vi "Cycle_Diag_Table_Read_TL24.vi"(7 "ERD Data In":T3[](array[typedef]) {"ERD Number" format="%.0x"}, 11 "error in (no error)":errorcluster) -> (2 "Cycle Buffer Status":T2, 3 "Diag Cycle String Out":string[][](array[string]), 8 "Cycle  Diag Array Out":T1[](array[typedef]), 15 "error out":errorcluster)   [LabVIEW 2016]
uses:
  Common/LabVIEW GEA2 Toolkit/LabVIEW_GEA2_Toolkit.lvlibp/type defs/ERD Read Data Out.ctl
  type defs/Cycle_Diag_Buffer_Status.ctl
  type defs/Cycle_Diag.ctl
  Common/LabVIEW GEA2 Toolkit/LabVIEW_GEA2_Toolkit.lvlibp
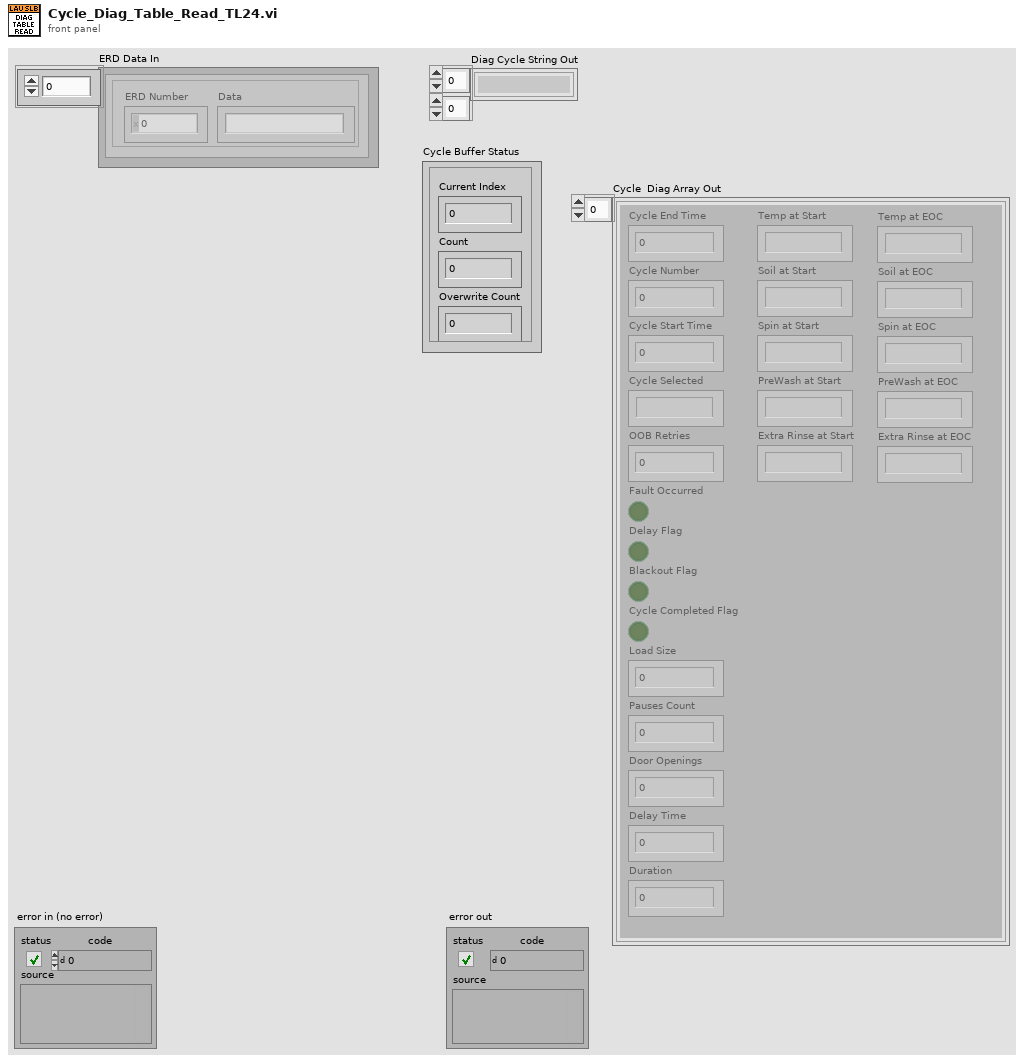
[diagram p1: front panel]
types:
  T1 = typedef "Cycle_Diag.ctl" = cluster{"Cycle End Time":u32, "Cycle Number":u32, "Cycle Start Time":u32, "OOB Retries":u8, "Temp at Start":string, "Soil at Start":string, "PreWash at Start":string, "Extra Rinse at Start":string, "Pauses Count":u8, "Fault Occurred":bool, "Delay Flag":bool, "Blackout Flag":bool, "Cycle Completed Flag":bool, "Temp at EOC":string, "Soil at EOC":string, "PreWash at EOC":string, "Extra Rinse at EOC":string, "Load Size":u8, "Door Openings":u8, "Cycle Selected":string, "Spin at Start":string, "Spin at EOC":string, "Delay Time":u16, "Duration":dbl}
  T2 = typedef "Cycle_Diag_Buffer_Status.ctl" = cluster{"Current Index":u16, "Count":u16, "Overwrite Count":u16}
  T3 = typedef "LabVIEW_GEA2_Toolkit.lvlibp/ERD Read Data Out.ctl" = cluster{"ERD Number":u16, "Data":string}
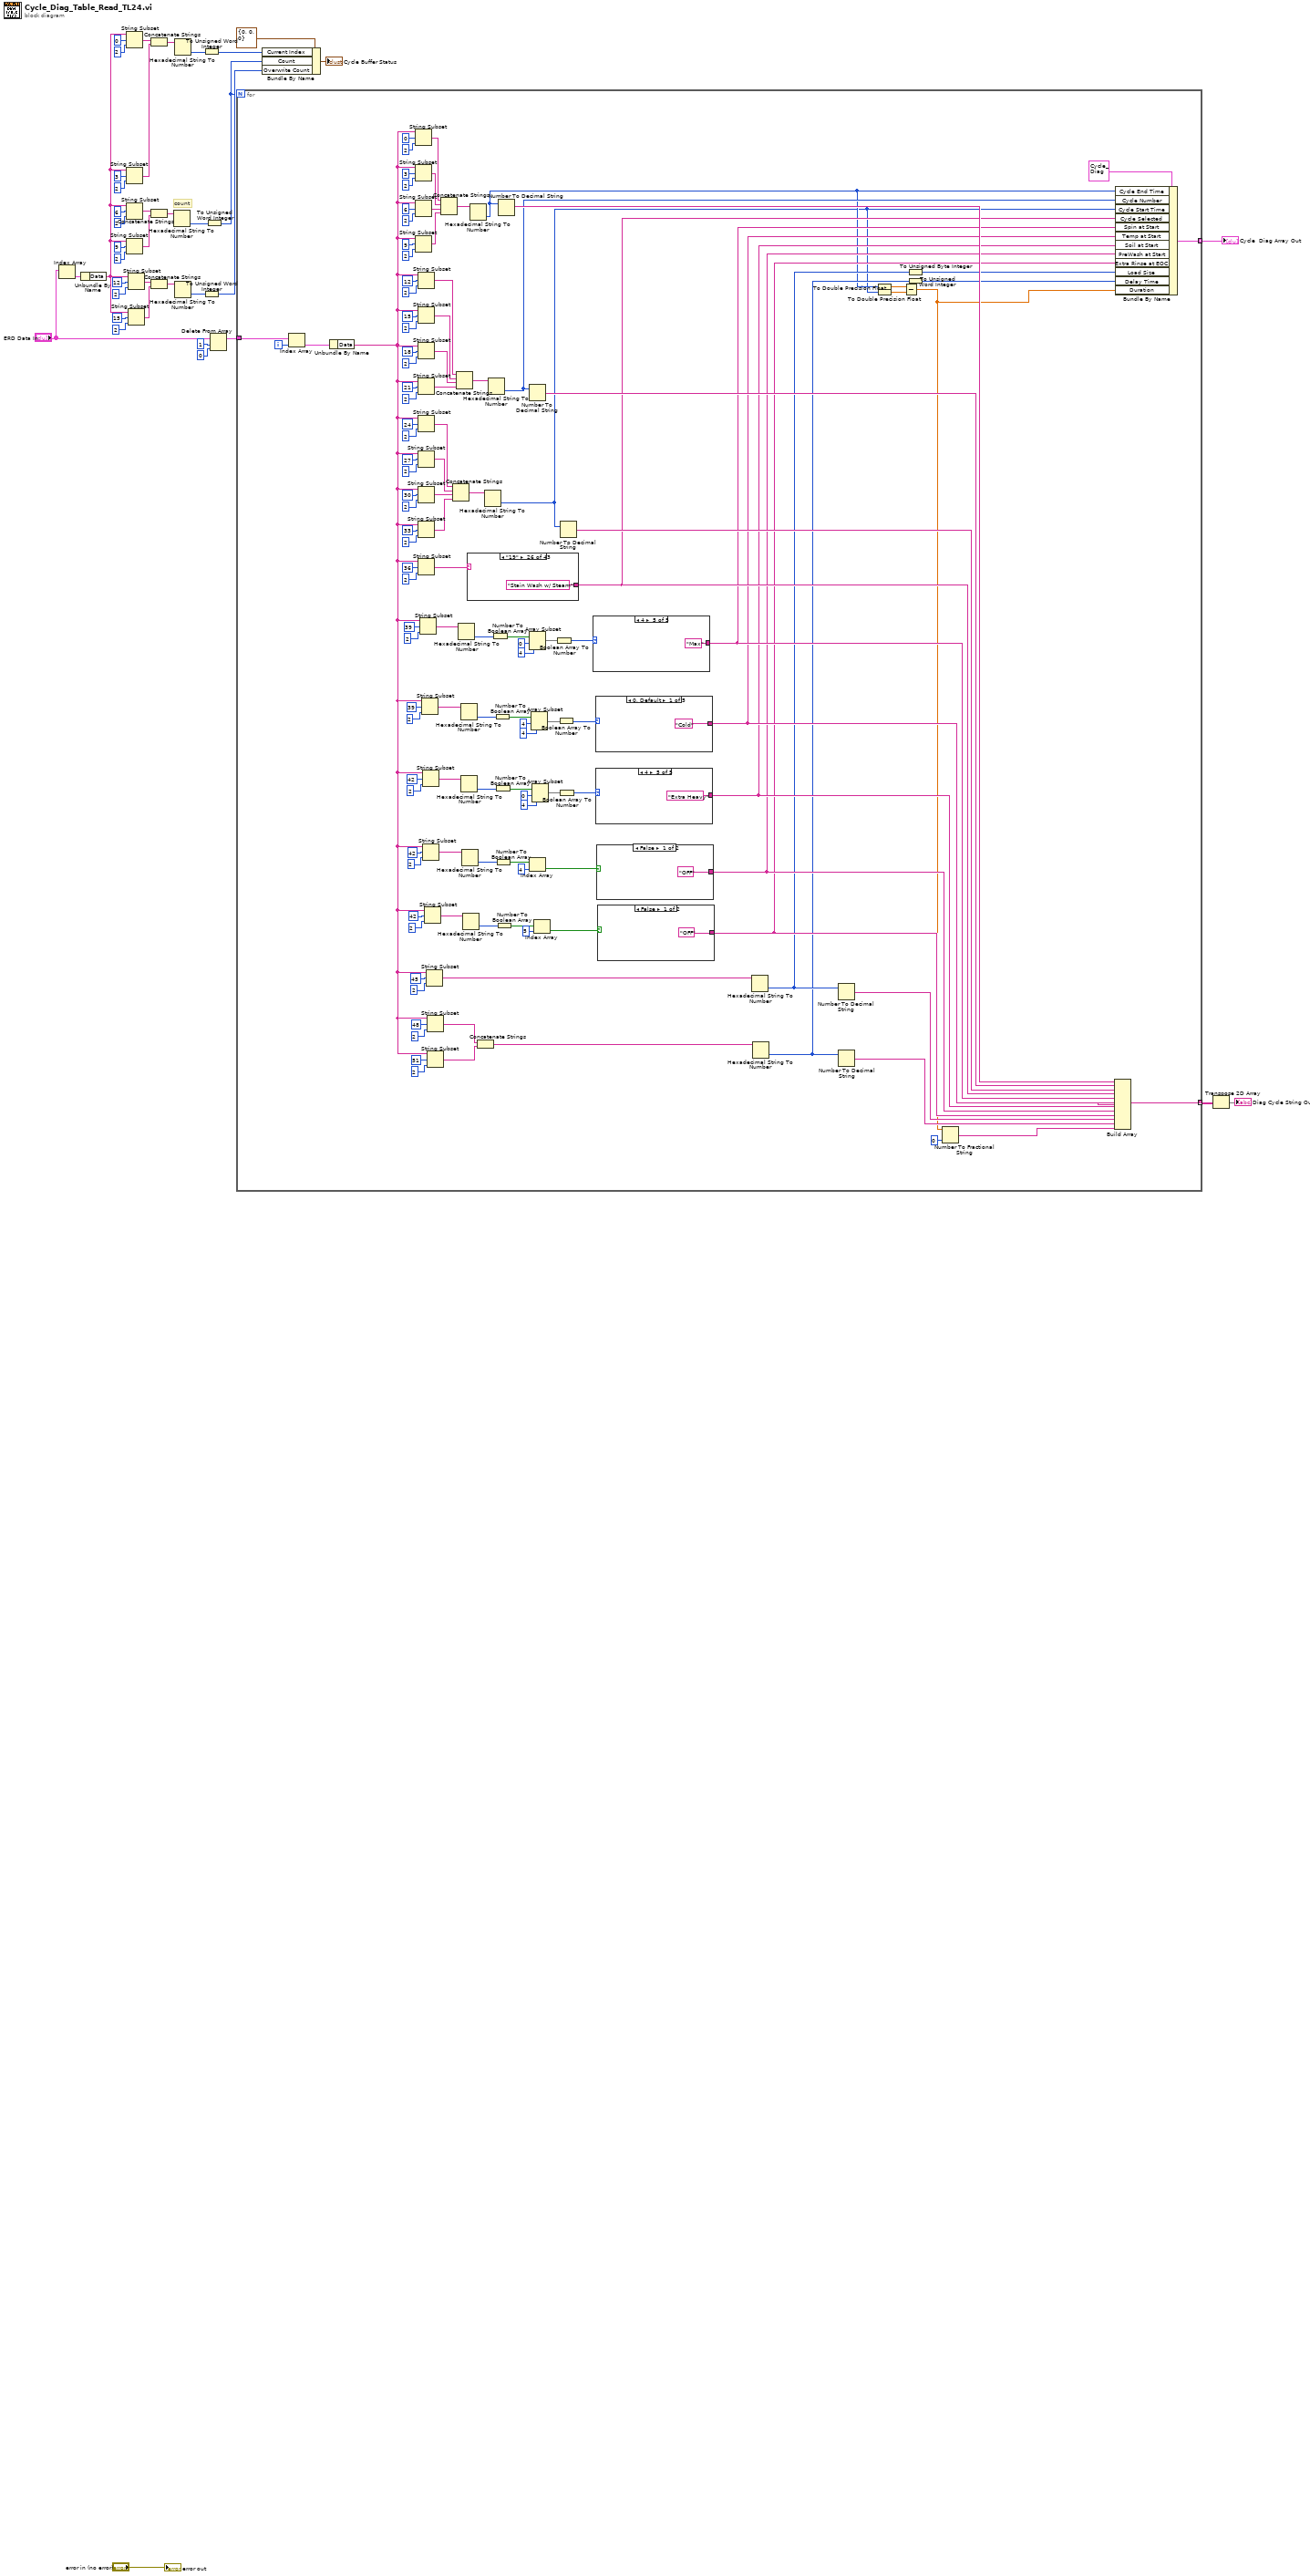
[diagram p0: block diagram]
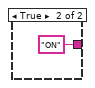
[diagram p2: hidden frame]
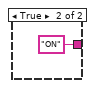
[diagram p3: hidden frame]
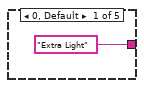
[diagram p4: hidden frame]
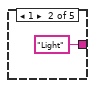
[diagram p5: hidden frame]
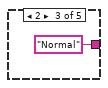
[diagram p6: hidden frame]
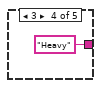
[diagram p7: hidden frame]
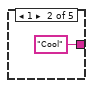
[diagram p8: hidden frame]
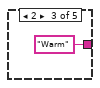
[diagram p9: hidden frame]
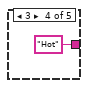
[diagram p10: hidden frame]
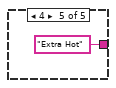
[diagram p11: hidden frame]
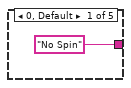
[diagram p12: hidden frame]
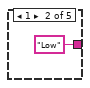
[diagram p13: hidden frame]
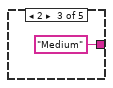
[diagram p14: hidden frame]
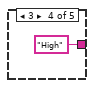
[diagram p15: hidden frame]
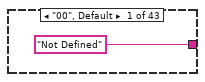
[diagram p16: hidden frame]
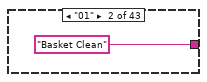
[diagram p17: hidden frame]
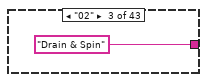
[diagram p18: hidden frame]
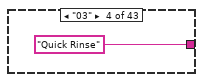
[diagram p19: hidden frame]
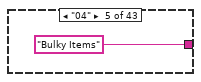
[diagram p20: hidden frame]
diagram:
  # "count"
  n1 = Index Array(array="ERD Data In") -> (element=w32:T3)  [unwired: 1 in]
  n2 = Unbundle By Name(w32) -> ("Data"=w12:string)
  n3 = String Subset(string=w12, offset (0)=0, length (rest)=2 ("length (rest)")) -> (substring=w21:string)
  n4 = String Subset(string=w12, offset (0)=3, length (rest)=2 ("length (rest)")) -> (substring=w22:string)
  n5 = String Subset(string=w12, offset (0)=6, length (rest)=2 ("length (rest)")) -> (substring=w36:string)
  n6 = String Subset(string=w12, offset (0)=9, length (rest)=2 ("length (rest)")) -> (substring=w35:string)
  n7 = String Subset(string=w12, offset (0)=12, length (rest)=2 ("length (rest)")) -> (substring=w23:string)
  n8 = String Subset(string=w12, offset (0)=15, length (rest)=2 ("length (rest)")) -> (substring=w24:string)
  n9 = Concatenate Strings(w21, w22) -> (w25:string)
  n10 = Concatenate Strings(w36, w35) -> (w34:string)
  n11 = Concatenate Strings(w23, w24) -> (w26:string)
  n12 = Hexadecimal String To Number(string=w34) -> (number=w33:u32)  [unwired: 2 in, 1 out]
  n13 = Hexadecimal String To Number(string=w25) -> (number=w27:u32)  [unwired: 2 in, 1 out]
  n14 = Hexadecimal String To Number(string=w26) -> (number=w28:u32)  [unwired: 2 in, 1 out]
  n15 = To Unsigned Word Integer(number=w27) -> (unsigned 16bit integer=w29:u16)
  n16 = To Unsigned Word Integer(number=w28) -> (unsigned 16bit integer=w30:u16)
  n17 = To Unsigned Word Integer(number=w33) -> (unsigned 16bit integer=w11:u16)
  n18 = Delete From Array(array="ERD Data In", length=1, index=0) -> (array with subset deleted=w8:T3[])  [unwired: 1 out]
  n19 = for {
    N: w11 -> [_]
    tunnel: w8 -> [w121]
    tunnel: [w118] -> w4 mode=indexing
    tunnel: [w117] -> w3 mode=indexing
    i -> [w120]
    n20 = Index Array(array=w121, index=w120) -> (element=w119:T3)
    n21 = Unbundle By Name(w119) -> ("Data"=w54:string)
    n22 = String Subset(string=w54, offset (0)=0, length (rest)=2 ("length (rest)")) -> (substring=w136:string)
    n23 = String Subset(string=w54, offset (0)=3, length (rest)=2 ("length (rest)")) -> (substring=w135:string)
    n24 = String Subset(string=w54, offset (0)=6, length (rest)=2 ("length (rest)")) -> (substring=w134:string)
    n25 = String Subset(string=w54, offset (0)=9, length (rest)=2 ("length (rest)")) -> (substring=w133:string)
    n26 = String Subset(string=w54, offset (0)=12, length (rest)=2 ("length (rest)")) -> (substring=w131:string)
    n27 = String Subset(string=w54, offset (0)=15, length (rest)=2 ("length (rest)")) -> (substring=w130:string)
    n28 = String Subset(string=w54, offset (0)=18, length (rest)=2 ("length (rest)")) -> (substring=w129:string)
    n29 = String Subset(string=w54, offset (0)=21, length (rest)=2 ("length (rest)")) -> (substring=w128:string)
    n30 = String Subset(string=w54, offset (0)=24, length (rest)=2 ("length (rest)")) -> (substring=w126:string)
    n31 = String Subset(string=w54, offset (0)=27, length (rest)=2 ("length (rest)")) -> (substring=w125:string)
    n32 = String Subset(string=w54, offset (0)=30, length (rest)=2 ("length (rest)")) -> (substring=w124:string)
    n33 = String Subset(string=w54, offset (0)=33, length (rest)=2 ("length (rest)")) -> (substring=w123:string)
    n34 = String Subset(string=w54, offset (0)=36, length (rest)=2 ("length (rest)")) -> (substring=w111:string)
    n35 = String Subset(string=w54, offset (0)=39, length (rest)=2 ("length (rest)")) -> (substring=w107:string)
    n36 = String Subset(string=w54, offset (0)=39, length (rest)=2 ("length (rest)")) -> (substring=w93:string)
    n37 = String Subset(string=w54, offset (0)=42, length (rest)=2 ("length (rest)")) -> (substring=w87:string)
    n38 = String Subset(string=w54, offset (0)=42, length (rest)=2 ("length (rest)")) -> (substring=w78:string)
    n39 = String Subset(string=w54, offset (0)=42, length (rest)=2 ("length (rest)")) -> (substring=w72:string)
    n40 = String Subset(string=w54, offset (0)=45, length (rest)=2 ("length (rest)")) -> (substring=w63:string)
    n41 = String Subset(string=w54, offset (0)=48, length (rest)=2 ("length (rest)")) -> (substring=w53:string)
    n42 = String Subset(string=w54, offset (0)=51, length (rest)=2 ("length (rest)")) -> (substring=w52:string)
    n43 = Concatenate Strings(w136, w135, w134, w133) -> (w132:string)
    n44 = Concatenate Strings(w126, w125, w124, w123) -> (w122:string)
    n45 = Concatenate Strings(w131, w130, w129, w128) -> (w127:string)
    n46 = Hexadecimal String To Number(string=w107) -> (number=w106:u32)  [unwired: 2 in, 1 out]
    n47 = Hexadecimal String To Number(string=w93) -> (number=w94:u32)  [unwired: 2 in, 1 out]
    n48 = Hexadecimal String To Number(string=w87) -> (number=w86:u32)  [unwired: 2 in, 1 out]
    n49 = Hexadecimal String To Number(string=w78) -> (number=w79:u32)  [unwired: 2 in, 1 out]
    n50 = Hexadecimal String To Number(string=w72) -> (number=w71:u32)  [unwired: 2 in, 1 out]
    n51 = case shown="\"19\"" w111 {
      tunnel: ["Not Defined" "Basket Clean" "Drain & Spin" "Quick Rinse" "Bulky Items" "Sanitize" "Towels & Sheets" "Steam Refresh" "Normal/Mixed" "Whites" "Dark Colors" "Jeans" "Hand Wash" "Delicates" "Speed Wash" "Heavy Duty" "Allergen" "Power Clean" "Rinse & Spin" "Single Item" "Colors" "Cold Wash" "Water on Demand" "Tub Clean" "Casuals w/ Steam" "Stain Wash w/ Steam" "Cottons" "Easy Care" "Active Wear" "Timed Dry" "Dewrinkle" "Air Fluff" "Steam Refresh" "Steam Dewrinkle" "Speed Dry" "Mixed" "Quick Dry" "Casuals" "Warm Up" "Energy Saver" "Antibacterial" "Rack Dry" "Baby Care"] -> w110
      frame "00", Default {
      }
      frame "01" {
      }
      frame "02" {
      }
      frame "03" {
      }
      frame "04" {
      }
      frame "05" {
      }
      frame "06" {
      }
      frame "07" {
      }
      frame "08" {
      }
      frame "09" {
      }
      frame "0A" {
      }
      frame "0B" {
      }
      frame "0C" {
      }
      frame "0D" {
      }
      frame "0E" {
      }
      frame "0F" {
      }
      frame "10" {
      }
      frame "11" {
      }
      frame "12" {
      }
      frame "13" {
      }
      frame "14" {
      }
      frame "15" {
      }
      frame "16" {
      }
      frame "17" {
      }
      frame "18" {
      }
      frame "19" {
      }
      frame "80" {
      }
      frame "81" {
      }
      frame "82" {
      }
      frame "83" {
      }
      frame "84" {
      }
      frame "85" {
      }
      frame "86" {
      }
      frame "87" {
      }
      frame "88" {
      }
      frame "89" {
      }
      frame "8A" {
      }
      frame "8B" {
      }
      frame "8C" {
      }
      frame "8D" {
      }
      frame "8E" {
      }
      frame "8F" {
      }
      frame "90" {
      }
    }
    n52 = Hexadecimal String To Number(string=w132) -> (number=w46:u32)  [unwired: 2 in, 1 out]
    n53 = Concatenate Strings(w53, w52) -> (w51:string)
    n54 = Hexadecimal String To Number(string=w122) -> (number=w45:u32)  [unwired: 2 in, 1 out]
    n55 = Hexadecimal String To Number(string=w127) -> (number=w113:u32)  [unwired: 2 in, 1 out]
    n56 = Number To Boolean Array(number=w106) -> (Boolean array=w105:bool[])
    n57 = Number To Boolean Array(number=w94) -> (Boolean array=w95:bool[])
    n58 = Number To Boolean Array(number=w86) -> (Boolean array=w85:bool[])
    n59 = Number To Boolean Array(number=w79) -> (Boolean array=w67:bool[])
    n60 = Number To Boolean Array(number=w71) -> (Boolean array=w70:bool[])
    n61 = Number To Decimal String(number=w46) -> (decimal integer string=w115:string)  [unwired: 1 in]
    n62 = Number To Decimal String(number=w113) -> (decimal integer string=w114:string)  [unwired: 1 in]
    n63 = Array Subset(array=w105, index=0, length=4) -> (w102:bool[])
    n64 = Index Array(array=w67, index=4) -> (element=w66:bool)
    n65 = Array Subset(array=w95, index=4, length=4) -> (w98:bool[])
    n66 = Array Subset(array=w85, index=0, length=4) -> (w82:bool[])
    n67 = Index Array(array=w70, index=5) -> (element=w65:bool)
    n68 = Boolean Array To Number(Boolean array=w102) -> (number=w101:u32)
    n69 = Boolean Array To Number(Boolean array=w98) -> (number=w99:u32)
    n70 = Boolean Array To Number(Boolean array=w82) -> (number=w81:u32)
    n71 = Number To Decimal String(number=w45) -> (decimal integer string=w112:string)  [unwired: 1 in]
    n72 = case shown="4" w101 {
      tunnel: ["No Spin" "Low" "Medium" "High" "Max"] -> w100
      frame 0, Default {
      }
      frame 1 {
      }
      frame 2 {
      }
      frame 3 {
      }
      frame 4 {
      }
    }
    n73 = case shown="0, Default" w99 {
      tunnel: ["Cold" "Cool" "Warm" "Hot" "Extra Hot"] -> w90
      frame 0, Default {
      }
      frame 1 {
      }
      frame 2 {
      }
      frame 3 {
      }
      frame 4 {
      }
    }
    n74 = case shown="4" w81 {
      tunnel: ["Extra Light" "Light" "Normal" "Heavy" "Extra Heavy"] -> w80
      frame 0, Default {
      }
      frame 1 {
      }
      frame 2 {
      }
      frame 3 {
      }
      frame 4 {
      }
    }
    n75 = case shown="False" w66 {
      tunnel: ["OFF" "ON"] -> w75
      frame False {
      }
      frame True {
      }
    }
    n76 = case shown="False" w65 {
      tunnel: ["OFF" "ON"] -> w64
      frame False {
      }
      frame True {
      }
    }
    n77 = Hexadecimal String To Number(string=w63) -> (number=w59:u32)  [unwired: 2 in, 1 out]
    n78 = Hexadecimal String To Number(string=w51) -> (number=w48:u32)  [unwired: 2 in, 1 out]
    n79 = Number To Decimal String(number=w59) -> (decimal integer string=w60:string)  [unwired: 1 in]
    n80 = Number To Decimal String(number=w48) -> (decimal integer string=w50:string)  [unwired: 1 in]
    n81 = To Double Precision Float(number=w46) -> (double precision float=w44:dbl)
    n82 = To Double Precision Float(number=w45) -> (double precision float=w43:dbl)
    n83 = Subtract(x=w44, y=w43) -> (x-y=w41:dbl)
    n84 = To Unsigned Byte Integer(number=w59) -> (unsigned 8bit integer=w49:u8)
    n85 = To Unsigned Word Integer(number=w48) -> (unsigned 16bit integer=w47:u16)
    n86 = Number To Fractional String(number=w41, precision (6)=i16 0) -> (F-format string=w42:string)  [unwired: 2 in]
    n87 = Build Array(w115, w114, w112, w110, w100, w90, w80, w75, w64, w60, w50, w42) -> (w117:string[])
    n88 = Bundle By Name(cluster=T1 {"Cycle End Time"=0, "Cycle Number"=0, "Cycle Start Time"=0, "OOB Retries"=0, "Temp at Start"="", "Soil at Start"="", "PreWash at Start"="", "Extra Rinse at Start"="", "Pauses Count"=0, "Fault Occurred"=FALSE, "Delay Flag"=FALSE, "Blackout Flag"=FALSE, "Cycle Completed Flag"=FALSE, "Temp at EOC"="", "Soil at EOC"="", "PreWash at EOC"="", "Extra Rinse at EOC"="", "Load Size"=0, "Door Openings"=0, "Cycle Selected"="", "Spin at Start"="", "Spin at EOC"="", "Delay Time"=0, "Duration"=0.0} ("Cycle History Diagnostics"), "Cycle End Time"=w46, "Cycle Number"=w113, "Cycle Start Time"=w45, "Cycle Selected"=w110, "Spin at Start"=w100, "Temp at Start"=w90, "Soil at Start"=w80, "PreWash at Start"=w75, "Extra Rinse at EOC"=w64, "Load Size"=w49, "Delay Time"=w47, "Duration"=w41) -> (w118:T1)
  }
  "Cycle  Diag Array Out" <- w4
  n89 = Bundle By Name(cluster=T2 {"Current Index"=0, "Count"=0, "Overwrite Count"=0} ("Cycle Buffer Status"), "Current Index"=w29, "Count"=w11, "Overwrite Count"=w30) -> (→"Cycle Buffer Status":T2)
  n90 = Transpose 2D Array(2D array=w3) -> (transposed array=→"Diag Cycle String Out":string[][])
  "error out" <- "error in (no error)"
